vi "PowerMap.vi"() -> ()   [LabVIEW 2012]
panel:
  in  "Dichroic - RJ T 473nm":dbl=0.75
  out "P (mW) Fiber":dbl
  out "Fiber T":dbl=inf
  out "P (mW) 532nm T":dbl
  out "P (mW) 473nm T":dbl=18.925524693104034
  out "P (mW) ThorLabs S121C":dbl=10.0
  in  "Dichroic - RJ T 532nm":dbl=0.75
  in  "Vo 473nm":dbl
  out "P (mW) 532nm R":dbl
  out "P (mW) 473nm R":dbl=1.6456977994003508
  in  "Vo 532nm":dbl
  # "532nm"
  # "437nm"
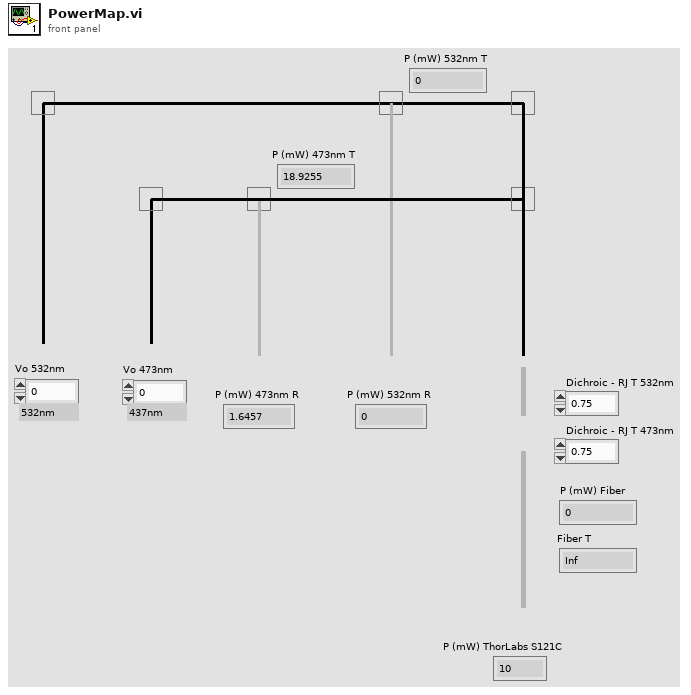
[diagram p1: front panel]
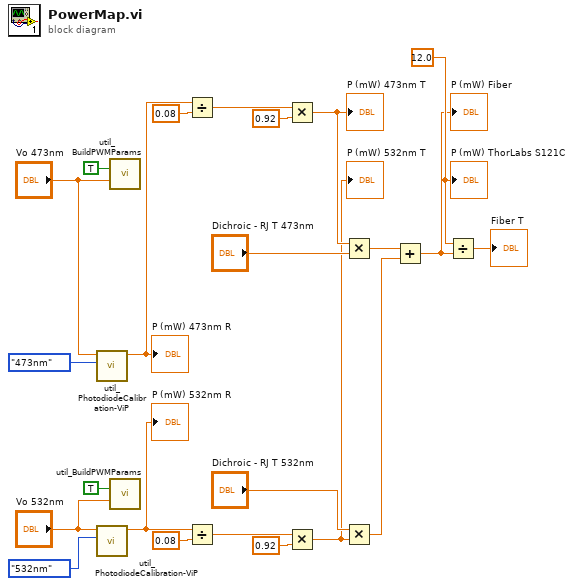
[diagram p0: block diagram]
diagram:
  w3 = 12.0 ("Power (mW) ThorLabs S121C")
  n1 = call "util_PhotodiodeCalibration-ViP.vi"("Enum"=enum16{"473nm", "532nm"}."473nm", "Vi"="Vo 473nm") -> ("P (mW)"=w9:dbl)  [unwired: 9 in]
  "P (mW) 473nm R" <- w9
  n2 = call "util_PhotodiodeCalibration-ViP.vi"("Enum"=enum16{"473nm", "532nm"}."532nm", "Vi"="Vo 532nm") -> ("P (mW)"=w8:dbl)  [unwired: 9 in]
  "P (mW) 532nm R" <- w8
  n3 = call "util_BuildPWMParams.vi"("Continous"=TRUE, "Amplitude (V)"="Vo 473nm") -> ()  [unwired: 13 in, 1 out]
  n4 = call "util_BuildPWMParams.vi"("Continous"=TRUE, "Amplitude (V)"="Vo 532nm") -> ()  [unwired: 13 in, 1 out]
  n5 = Divide(x=w9, y=0.08) -> (x/y=w14:dbl)
  n6 = Divide(x=w8, y=0.08) -> (x/y=w17:dbl)
  n7 = Multiply(x=w14, y=0.92) -> (x*y=w11:dbl)
  "P (mW) 473nm T" <- w11
  n8 = Multiply(x=w17, y=0.92) -> (x*y=w6:dbl)
  "P (mW) 532nm T" <- w6
  n9 = Multiply(x=w11, y="Dichroic - RJ T 473nm") -> (x*y=w5:dbl)
  n10 = Multiply(x="Dichroic - RJ T 532nm", y=w6) -> (x*y=w4:dbl)
  n11 = Add(x=w5, y=w4) -> (x+y=w2:dbl)
  "P (mW) Fiber" <- w2
  n12 = Divide(x=w3, y=w2) -> (x/y=→"Fiber T":dbl)
  "P (mW) ThorLabs S121C" <- w3
